vi "MultiNPointAverager.vi"(7 "N point average":i32, 11 "Array of values":dbl[](array[numeric])) -> (3 "Array of averages":dbl[](array[numeric]))   [LabVIEW 2012]
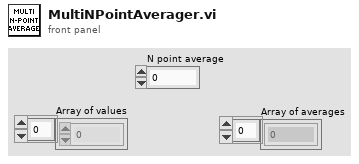
[diagram p1: front panel]
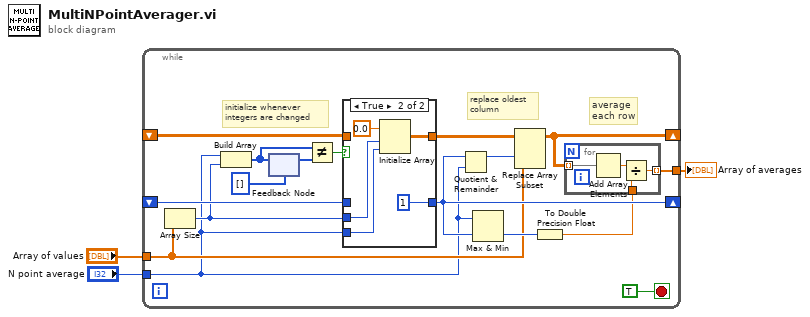
[diagram p0: block diagram]
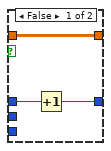
[diagram p2: hidden frame]
diagram:
  n1 = while {
    tunnel: [w19] -> w3
    tunnel: "Array of values" -> [w11]
    tunnel: "N point average" -> [w9]
    shift-right: [w16] -> _
    shift-left: _ -> [w14]
    shift-right: [w13] -> _
    shift-left: _ -> [w12]
    stop <- TRUE stop-if-true
    # "average\neach row"
    # "initialize whenever\nintegers are changed"
    # "replace oldest\ncolumn"
    n2 = Array Size(array=w11) -> (size(s)=w10:i32)
    n3 = Build Array(w9, w10) -> (w7:i32[])
    n4 = feedback-in #1(w7) -> ()
    n5 = feedback #1(i32[] []) -> (w8:i32[])
    n6 = Not Equal?(x=w7, y=w8) -> (x != y?=w6:bool)
    n7 = case shown="True" w6 {
      tunnel: [w23 w26] -> w15
      tunnel: w14 -> [w23 _]
      tunnel: [w21 1] -> w13
      tunnel: w12 -> [w22 _]
      tunnel: w10 -> [_ w25]
      tunnel: w9 -> [_ w24]
      frame False {
        n8 = Increment(x=w22) -> (x+1=w21:i32)
      }
      frame True {
        n9 = Initialize Array(0.0 ("element"), w25, w24) -> (w26:dbl[][])
      }
    }
    n10 = Quotient & Remainder(x=w13, y=w9) -> (x-y*floor(x/y)=w20:i32)  [unwired: 1 out]
    n11 = Max & Min(x=w9, y=w13) -> (min(x,y)=w18:i32)  [unwired: 1 out]
    n12 = Replace Array Subset(array=w15, new element=w11, index (col)=w20) -> (w16:dbl[][])  [unwired: 1 in]
    n13 = To Double Precision Float(number=w18) -> (double precision float=w4:dbl)
    n14 = for {
      tunnel: w16 -> [w32] mode=indexing
      tunnel: w4 -> [w30]
      tunnel: [w29] -> w19 mode=indexing
      n15 = Add Array Elements(numeric array=w32) -> (sum=w31:dbl)
      n16 = Divide(x=w31, y=w30) -> (x/y=w29:dbl)
    }
  }
  "Array of averages" <- w3
